vi "Set_AppPaths.vi"(8 "error in":errorcluster, 11 "EVE in":refnum<class "EVE.lvclass">) -> (0 "error out":errorcluster, 3 "EVE out":refnum<class "EVE.lvclass">)   [LabVIEW 2013, in "EVE.lvclass"]
uses:
  EVE.lvclass
  EVE.lvclass/EVE.ctl
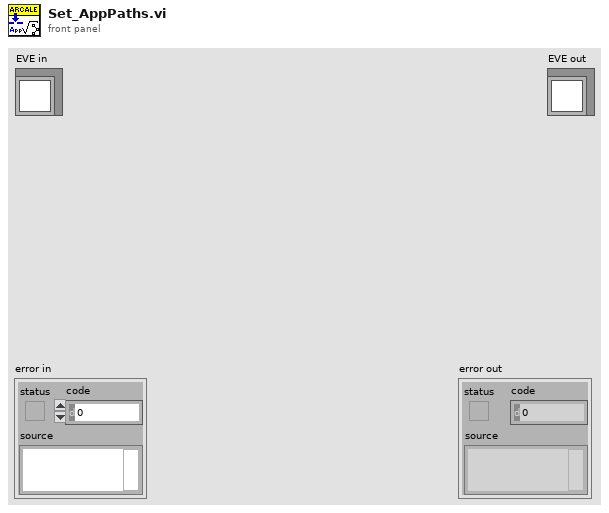
[diagram p1: front panel]
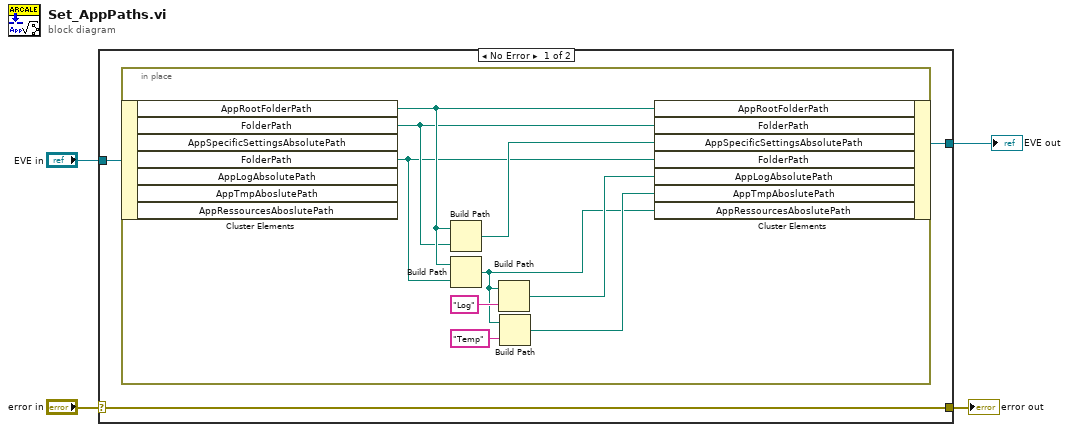
[diagram p0: block diagram]
diagram:
  n1 = case shown="No Error" "error in" {
    selector: "error in" -> [w6 w18]
    tunnel: [w6 w18] -> w3
    tunnel: [w5 w17] -> w1
    tunnel: "EVE in" -> [w7 w17]
    frame No Error {
      n2 = in-place {
        n3 = in-place-cluster #1(w7) -> ("AppRootFolderPath"=w11:path, "FolderPath"=w10:path, "FolderPath"=w9:path)  [unwired: 4 out]
        n4 = Build Path(base path=w11, name or relative path=w10) -> (appended path=w16:path)
        n5 = Build Path(base path=w11, name or relative path=w9) -> (appended path=w8:path)
        n6 = Build Path(base path=w8, name or relative path="Log") -> (appended path=w14:path)
        n7 = Build Path(base path=w8, name or relative path="Temp") -> (appended path=w12:path)
        n8 = in-place-cluster #1("AppRootFolderPath"=w11, "FolderPath"=w10, "AppSpecificSettingsAbsolutePath"=w16, "FolderPath"=w9, "AppLogAbsolutePath"=w14, "AppTmpAboslutePath"=w12, "AppRessourcesAboslutePath"=w8) -> (w5:refnum<class "EVE.lvclass">)
      }
    }
    frame Error {
    }
  }
  "error out" <- w3
  "EVE out" <- w1
